vi "AIT 1553 - Create Sysdef Tree from DB Bus Configuration.vi"(0 "Section Ref in":T1 format="%.0x", 1 "Called From SysDef API (F)":bool, 9 "Bus":T2, 11 "error in":errorcluster) -> (4 "Section Ref out":T1 format="%.0x", 6 "Item Ref":T1 format="%.0x", 15 "error out":errorcluster)   [LabVIEW 2013, in "AIT 1553 Custom Device.lvlib"]
uses:
  AIT 1553 Custom Device.lvlib
  <vilib>/NI Veristand/Custom Device API/Custom Device Item Ref.ctl
  Controls/1553_Bus.ctl
  Controls/1553_Bus_Controller.ctl
  Controls/1553_BC_Message.ctl
  Controls/1553 Param.ctl
  Controls/1553_Acyclic_Frame.ctl
  Controls/1553_Bus_Monitor.ctl
  Controls/1553_BM_Message.ctl
  Controls/1553_RT_Message.ctl
  <vilib>/NI Veristand/Custom Device Tools/Custom Device Utility Library/Search Direction.ctl
  Controls and Global/Global.vi
  <vilib>/NI Veristand/Custom Device Tools/Custom Device Utility Library/NI VeriStand - Search for Item by GUID.vi
  <vilib>/NI Veristand/Custom Device Tools/Custom Device Utility Library/Custom Device Utility Library.lvlib
  <vilib>/NI Veristand/Custom Device API/Custom Device API.lvlib
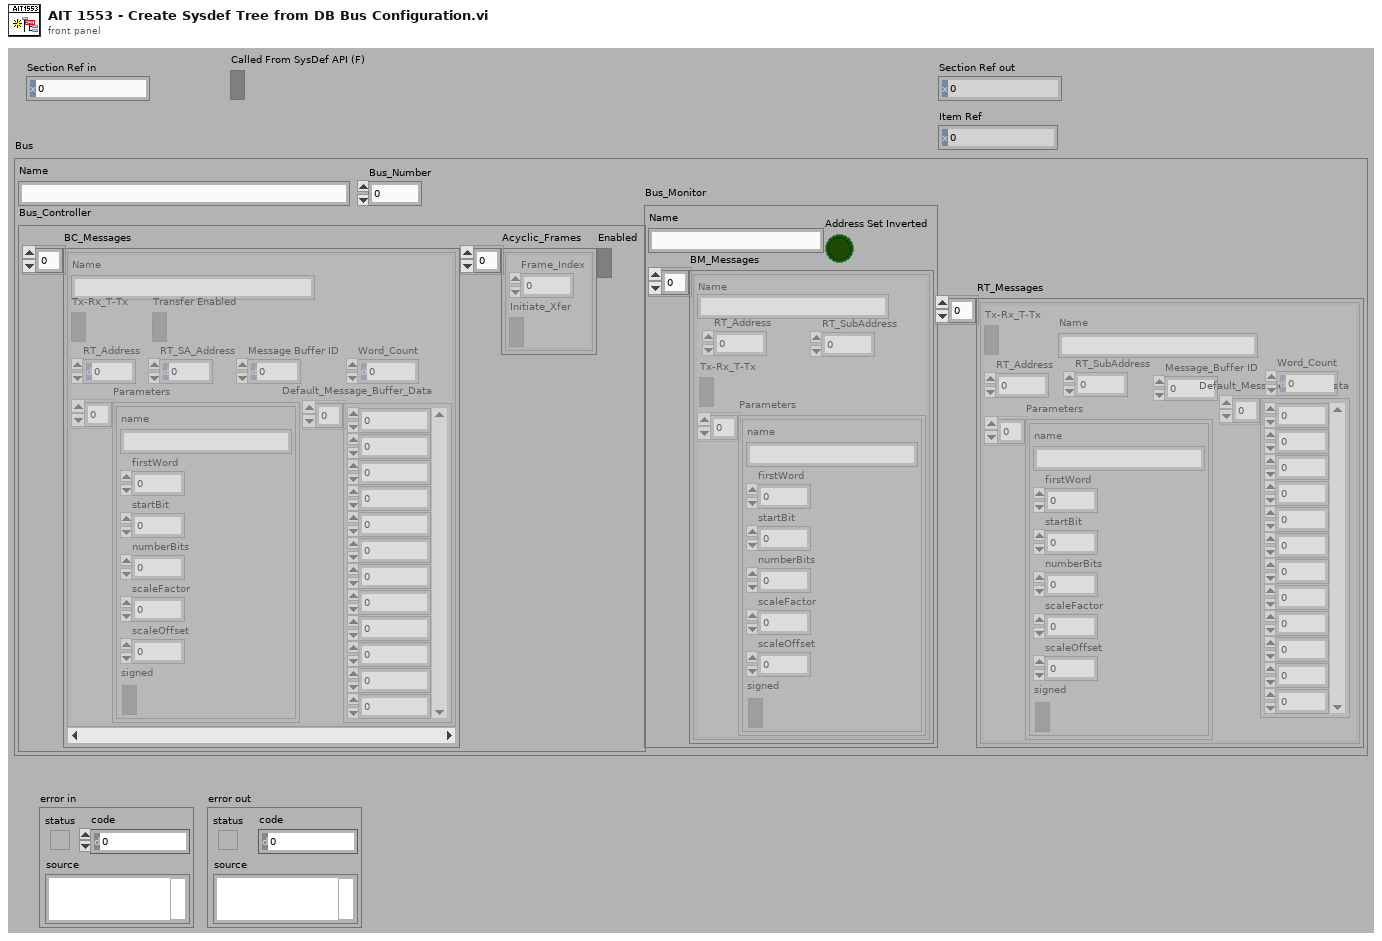
[diagram p1: front panel]
types:
  T1 = typedef "Custom Device API.lvlib/Custom Device Item Ref.ctl" = u64
  T2 = typedef "AIT 1553 Custom Device.lvlib/1553_Bus.ctl" = cluster{"Name":string, "Bus_Number":u8, "Bus_Controller":T3, "Bus_Monitor":T7, "RT_Messages":T9[]}
  T3 = typedef "AIT 1553 Custom Device.lvlib/1553_Bus_Controller.ctl" = cluster{"BC_Messages":T4[], "Acyclic_Frames":T6[], "Enabled":bool}
  T4 = typedef "AIT 1553 Custom Device.lvlib/1553_BC_Message.ctl" = cluster{"Name":string, "Tx-Rx_T-Tx":bool, "RT_Address":u8, "RT_SA_Address":u8, "Parameters":T5[], "Transfer Enabled":bool, "Message Buffer ID":u16, "Default_Message_Buffer_Data":u16[], "Word_Count":u8}
  T5 = typedef "AIT 1553 Custom Device.lvlib/1553 Param.ctl" = cluster{"name":string, "firstWord":i32, "startBit":i32, "numberBits":i32, "scaleFactor":dbl, "scaleOffset":dbl, "signed":bool}
  T6 = typedef "AIT 1553 Custom Device.lvlib/1553_Acyclic_Frame.ctl" = cluster{"Frame_Index":u8, "Initiate_Xfer":bool}
  T7 = typedef "AIT 1553 Custom Device.lvlib/1553_Bus_Monitor.ctl" = cluster{"Name":string, "BM_Messages":T8[], "Address Set Inverted":bool}
  T8 = typedef "AIT 1553 Custom Device.lvlib/1553_BM_Message.ctl" = cluster{"RT_Address":u8, "RT_SubAddress":u8, "Tx-Rx_T-Tx":bool, "Parameters":T5[], "Name":string}
  T9 = typedef "AIT 1553 Custom Device.lvlib/1553_RT_Message.ctl" = cluster{"RT_Address":u8, "RT_SubAddress":u8, "Tx-Rx_T-Tx":bool, "Parameters":T5[], "Message_Buffer ID":u16, "Default_Message_Buffer_Data":u16[], "Word_Count":u8, "Name":string}
  T10 = typedef "Custom Device Utility Library.lvlib/Search Direction.ctl" = enum16{"Down", "Up"}
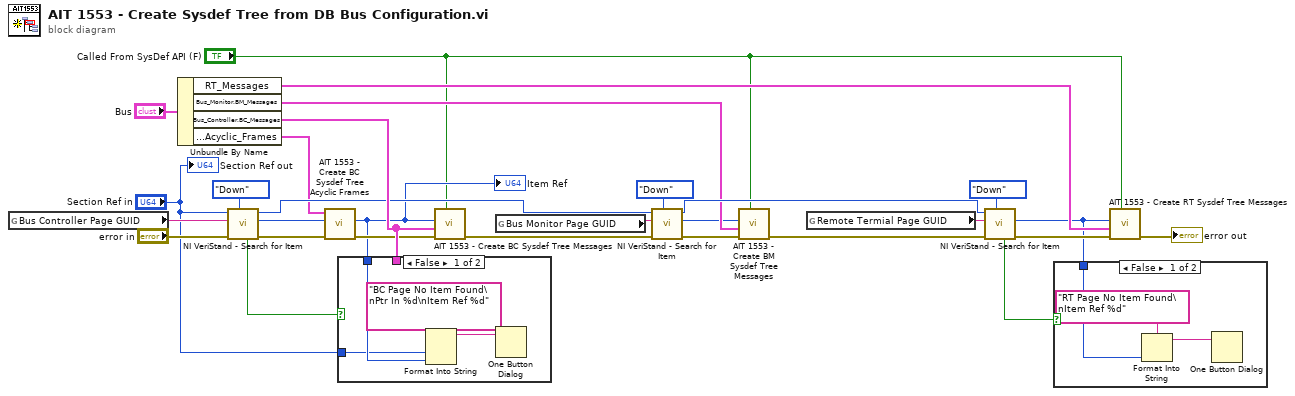
[diagram p0: block diagram]
diagram:
  n1 = global read "Global.vi" "Bus Controller Page GUID"() -> (w27:string)
  n2 = Unbundle By Name("Bus") -> ("RT_Messages"=w20:T9[], "Bus_Monitor.BM_Messages"=w11:T8[], "Bus_Controller.BC_Messages"=w24:T4[], "Bus_Controller.Acyclic_Frames"=w2:T6[])
  n3 = call-poly <vilib>:"NI VeriStand - Search for Item.vi"("Direction (Down)"=Search_Direction."Down", "error in"="error in", "Item GUID"=w27, "Section Ref in"="Section Ref in") -> ("error out"=w6:errorcluster, "Item Ref"=w3:T1, "Section Ref out"=w7:T1, "Found"=w25:bool)  [unwired: 4 in]
  n4 = call "AIT 1553 - Create BC Sysdef Tree Acyclic Frames.vi"("error in"=w6, "Section Ptr"=w3, "Acyclic_Frames"=w2) -> ("error out"=w5:errorcluster, "Section Ptr Out"=w4:T1)  [unwired: 7 in]
  "Item Ref" <- w4
  n5 = case shown="False" w25 {
    tunnel: w4 -> [w31 _]
    tunnel: w24 -> [_ _]
    tunnel: "Section Ref in" -> [w30 _]
    frame False {
      n6 = Format Into String(format string="BC Page No Item Found\nPtr In %d\nItem Ref %d" ("message"), w30, w31) -> (resulting string=w32:string)  [unwired: 2 in, 1 out]
      n7 = One Button Dialog(message=w32) -> ()  [unwired: 1 in, 1 out]
    }
    frame True {
    }
  }
  n8 = call "AIT 1553 - Create BC Sysdef Tree Messages.vi"("Called From SysDef API (F)"="Called From SysDef API (F)", "error in"=w5, "BC Messages"=w24, "Section Ptr"=w4) -> ("error out"=w13:errorcluster)  [unwired: 7 in]
  n9 = global read "Global.vi" "Bus Monitor Page GUID"() -> (w8:string)
  n10 = call-poly <vilib>:"NI VeriStand - Search for Item.vi"("Direction (Down)"=Search_Direction."Down", "error in"=w13, "Item GUID"=w8, "Section Ref in"=w7) -> ("error out"=w9:errorcluster, "Item Ref"=w10:T1, "Section Ref out"=w12:T1)  [unwired: 4 in, 1 out]
  n11 = call "AIT 1553 - Create BM Sysdef Tree Messages.vi"("Called From SysDef API (F)"="Called From SysDef API (F)", "error in"=w9, "BM Messages"=w11, "Section Ptr"=w10) -> ("error out"=w15:errorcluster)  [unwired: 7 in]
  n12 = global read "Global.vi" "Remote Termial Page GUID"() -> (w22:string)
  n13 = call-poly <vilib>:"NI VeriStand - Search for Item.vi"("Direction (Down)"=Search_Direction."Down", "error in"=w15, "Item GUID"=w22, "Section Ref in"=w12) -> ("error out"=w21:errorcluster, "Item Ref"=w17:T1, "Found"=w18:bool)  [unwired: 4 in, 1 out]
  n14 = case shown="False" w18 {
    tunnel: w17 -> [w35 _]
    frame False {
      n15 = Format Into String(format string="RT Page No Item Found\nItem Ref %d" ("message"), w35) -> (resulting string=w34:string)  [unwired: 2 in, 1 out]
      n16 = One Button Dialog(message=w34) -> ()  [unwired: 1 in, 1 out]
    }
    frame True {
    }
  }
  n17 = call "AIT 1553 - Create RT Sysdef Tree Messages.vi"("Called From SysDef API (F)"="Called From SysDef API (F)", "error in"=w21, "RT_Messages"=w20, "Section Ptr"=w17) -> ("error out"=→"error out":errorcluster)  [unwired: 7 in]
  "Section Ref out" <- "Section Ref in"
